vi "SSH Get .NET Refnum.vi"(8 "Error In":errorcluster, 11 "SSH Session":refnum<k1>) -> (0 "Error Out":errorcluster, 2 "SSH .NET Refnum":refnum<k24>, 3 "SSH Session":refnum<k1>)   [LabVIEW 2020, in "LMH-LINX.lvlib"]
uses:
  LMH-LINX.lvlib
  c:/p4/penguin/lvaddon/MakerHub/LINX/trunk/20.1/objects/MakerHub_LINX/win32U/i386/msvc90/release/LabVIEW/vi.lib/MakerHub/LINX/Resources/Renci.SshNet.dll
  Resources/Renci.SshNet.dll
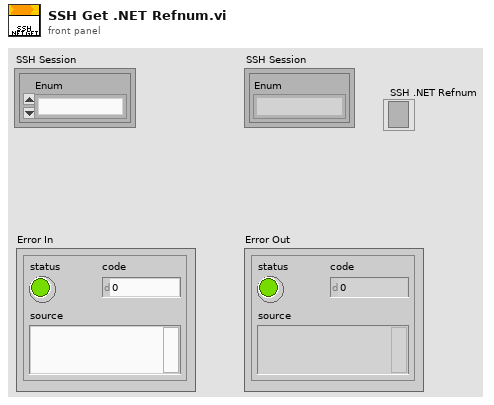
[diagram p1: front panel]
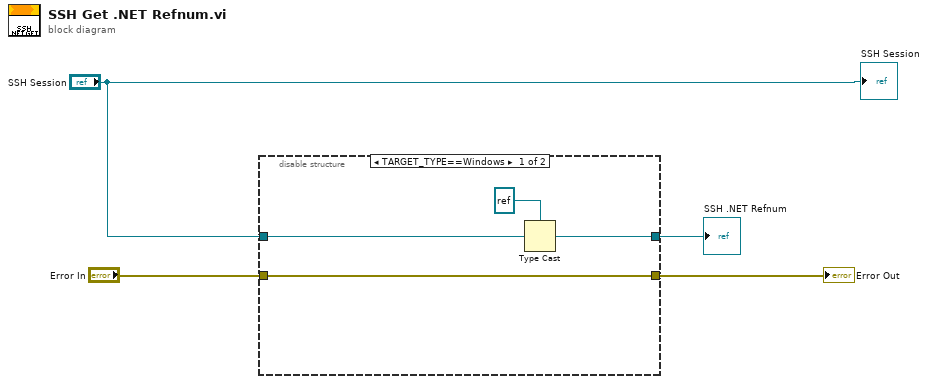
[diagram p0: block diagram]
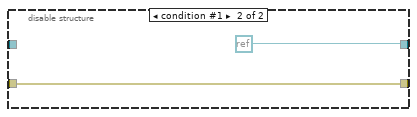
[diagram p2: hidden frame]
diagram:
  n1 = disable-structure shown="TARGET_TYPE==Windows" {
    disable-tunnel: [w7 w10] -> w3
    disable-tunnel: "Error In" -> [w7 w10]
    disable-tunnel: "SSH Session" -> [w8 _]
    disable-tunnel: [w6 refnum<k0> refnum] -> w1
    frame condition #0 (active) {
      n2 = Type Cast(type=refnum<k24> refnum ("SSH Session"), x=w8) -> (*(type *) &x=w6:refnum<k24>)
    }
    frame condition #1 {
    }
  }
  "Error Out" <- w3
  "SSH .NET Refnum" <- w1
  "SSH Session" <- "SSH Session"
